vi "dfd_DFXP negate (vv).vi"(9 "High 64":i64[](array[numeric]) format="%.0x", 10 "Low 64":u64[](array[numeric])) -> (1 "High 64":i64[](array[numeric]), 2 "Low 64":u64[](array[numeric]))   [LabVIEW 2017, in "NI_DigFilter_FXP.lvlib"]
uses:
  <vilib>/addons/Digital Filter Design/NI_DigFilter_FXP.lvlib
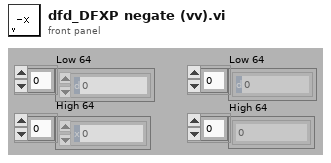
[diagram p1: front panel]
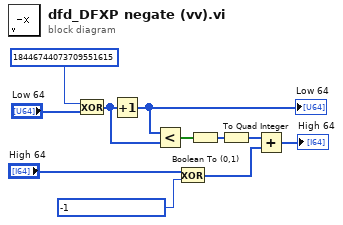
[diagram p0: block diagram]
diagram:
  n1 = Exclusive Or(1:"Low 64", 2:u64 18446744073709551615 ("y")) -> (0:w5:u64[])
  n2 = Increment(x=w5) -> (x+1=w3:u64[])
  "Low 64" <- w3
  n3 = Less?(x=w3, y=w5) -> (x < y?=w9:bool[])
  n4 = Exclusive Or(1:i64 -1 ("y"), 2:"High 64") -> (0:w7:i64[])
  n5 = Boolean To (0,1)(Boolean=w9) -> (0, 1=w8:i16[])
  n6 = To Quad Integer(1:w8) -> (0:w6:i64[])
  n7 = Add(x=w6, y=w7) -> (x+y=→"High 64":i64[])
